vi "initialise.vi"(8 "error in (no error)":errorcluster, 11 "GenericTrajectory in":refnum<class "TrajectoryDL121017Hopping.lvclass">) -> (0 "error out":errorcluster, 3 "GenericTrajectory out":refnum<class "TrajectoryDL121017Hopping.lvclass">)   [LabVIEW 2010, in "TrajectoryDL121017Hopping.lvclass"]
doc: "Calculates trajectory coordinates."
uses:
  TrajectoryDL121017Hopping.lvclass
  TrajectoryDL091126GenericVoxel/TrajectoryDL091126GenericVoxel/TrajectoryDL091126GenericVoxel.lvclass
panel:
  out "number of pixels":i32
  out "failed?":bool
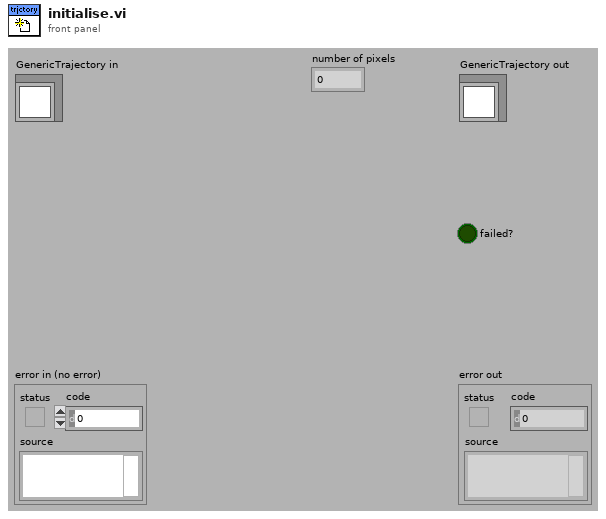
[diagram p1: front panel]
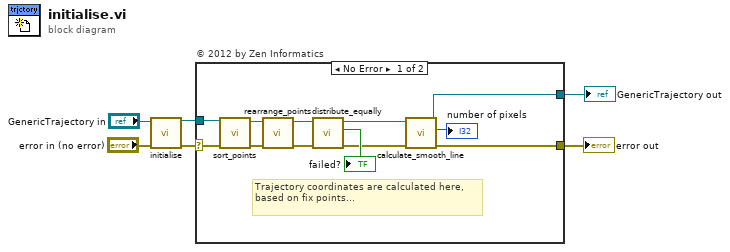
[diagram p0: block diagram]
diagram:
  n1 = call-parent "initialise.vi"("error in (no error)"="error in (no error)", "GenericTrajectory in"="GenericTrajectory in") -> ("error out"=w4:errorcluster, "GenericTrajectory out"=w3:refnum<class "TrajectoryDL121017Hopping.lvclass">)  [unwired: 8 in]
  n2 = case "© 2012 by Zen Informatics" shown="No Error" w4 {
    selector: w4 -> [w17 w19]
    tunnel: w3 -> [w15 w20]
    tunnel: [w9 w20] -> w2
    tunnel: [w7 w19] -> w1
    frame No Error {
      # "Trajectory coordinates are calculated here, based on fix points..."
      n3 = call "sort_points.vi"("error in (no error)"=w17, "TrajectoryDL121017Hopping in"=w15) -> ("error out"=w18:errorcluster, "TrajectoryDL121017Hopping out"=w16:refnum<class "TrajectoryDL121017Hopping.lvclass">)  [unwired: 8 in]
      n4 = call "rearrange_points.vi"("error in (no error)"=w18, "TrajectoryDL121017Hopping in"=w16) -> ("error out"=w11:errorcluster, "TrajectoryDL121017Hopping out"=w12:refnum<class "TrajectoryDL121017Hopping.lvclass">)  [unwired: 8 in]
      n5 = call-dynamic "distribute_equally.vi"("error in (no error)"=w11, "TrajectoryDL091126GenericVoxel in"=w12) -> ("error out"=w10:errorcluster, "failed?"=→"failed?":bool, "TrajectoryDL091126GenericVoxel out"=w8:refnum<class "TrajectoryDL121017Hopping.lvclass">)  [unwired: 7 in]
      n6 = call "calculate_smooth_line.vi"("error in (no error)"=w10, "TrajectoryDL121017Hopping in"=w8) -> ("error out"=w7:errorcluster, "number of pixels"=→"number of pixels":i32, "TrajectoryDL121017Hopping out"=w9:refnum<class "TrajectoryDL121017Hopping.lvclass">)  [unwired: 7 in]
    }
    frame Error {
    }
  }
  "error out" <- w1
  "GenericTrajectory out" <- w2
